vi "UI Main.vi"() -> ()   [LabVIEW 2020]
uses:
  controls/UI Data.ctl
  support/Message Queue/Message Cluster.ctl
  Globals/Global - All UI Loop Stop.vi
  Globals/Global - UI Stream and Variable Connections.vi
  Globals/Global - Configuration Options.vi
  support/User Event - Stop/User Event - Stop.lvlib
  support/Message Queue/Message Queue.lvlib
panel:
  in  "UI Error":string="UI Error"
  in  "Invalid Message Loop Message":string="The invalid message string \"%s\" was received in the Message Handling Loop."
  out "Current Logging State":u16(ring) items=["Logging", "Idle (Safe State)", "Unknown - Disconnected"]
  in  "Exit":bool
  out "System Status":string
  in  "Settings Tab":enum32{"UI Commands", "System Monitoring"}(tab)
  in  "Live Data Channel":u32 max=3 step=1
  out "Live Data":waveform(dbl)(graph)
  in  "Stop Live Data":bool
  in  "Acquire Live Data":bool
  out "Most recent manually-triggered log file":path
  in  "Force Trigger":bool
  out "Number of Data Files":u32
  out "Largest Contiguous Memory (bytes)":dbl(graph)
  out "Resource Utilization (%)":cluster{dbl, "Double":dbl, dbl}(graph)
  out "System Time":timestamp
  out "Connected?":bool
  in  "Connect to Controller":bool
  in  "Controller Address":string
  # "LabVIEW Real-Time Waveform Acquisition and Logging (NI-DAQmx)"
  # "Connection Settings"
  # "Live Data"
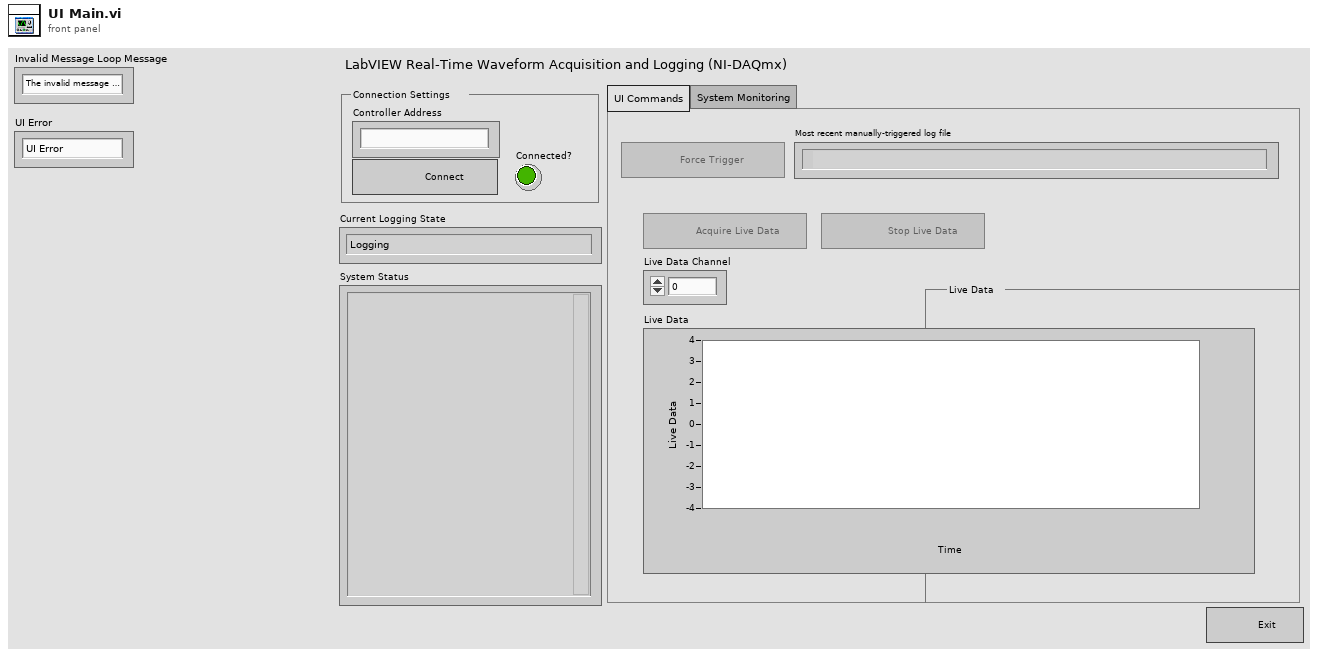
[diagram p1: front panel]
types:
  T1 = typedef "UI Data.ctl" = cluster{"Create Log File Ref":refnum<vi>, "Acquire Live Data Ref":refnum<vi>, "Stop Live Data Ref":refnum<vi>}
  T2 = typedef "Message Queue.lvlib/All Host Message Queues.ctl" = cluster{"UI":refnum<queue>}
  T3 = typedef "Message Queue.lvlib/Message Cluster.ctl" = cluster{"Message":string, "Message Data":variant}
  T4 = typedef "Variable References.ctl" = cluster{"CPU Usage":refnum<k21>, "Contiguous Memory":refnum<k21>, "Buffer Backlog":refnum<k21>, "Drive Space":refnum<k21>, "Number of Data Files":refnum<k21>, "System Time":refnum<k21>}
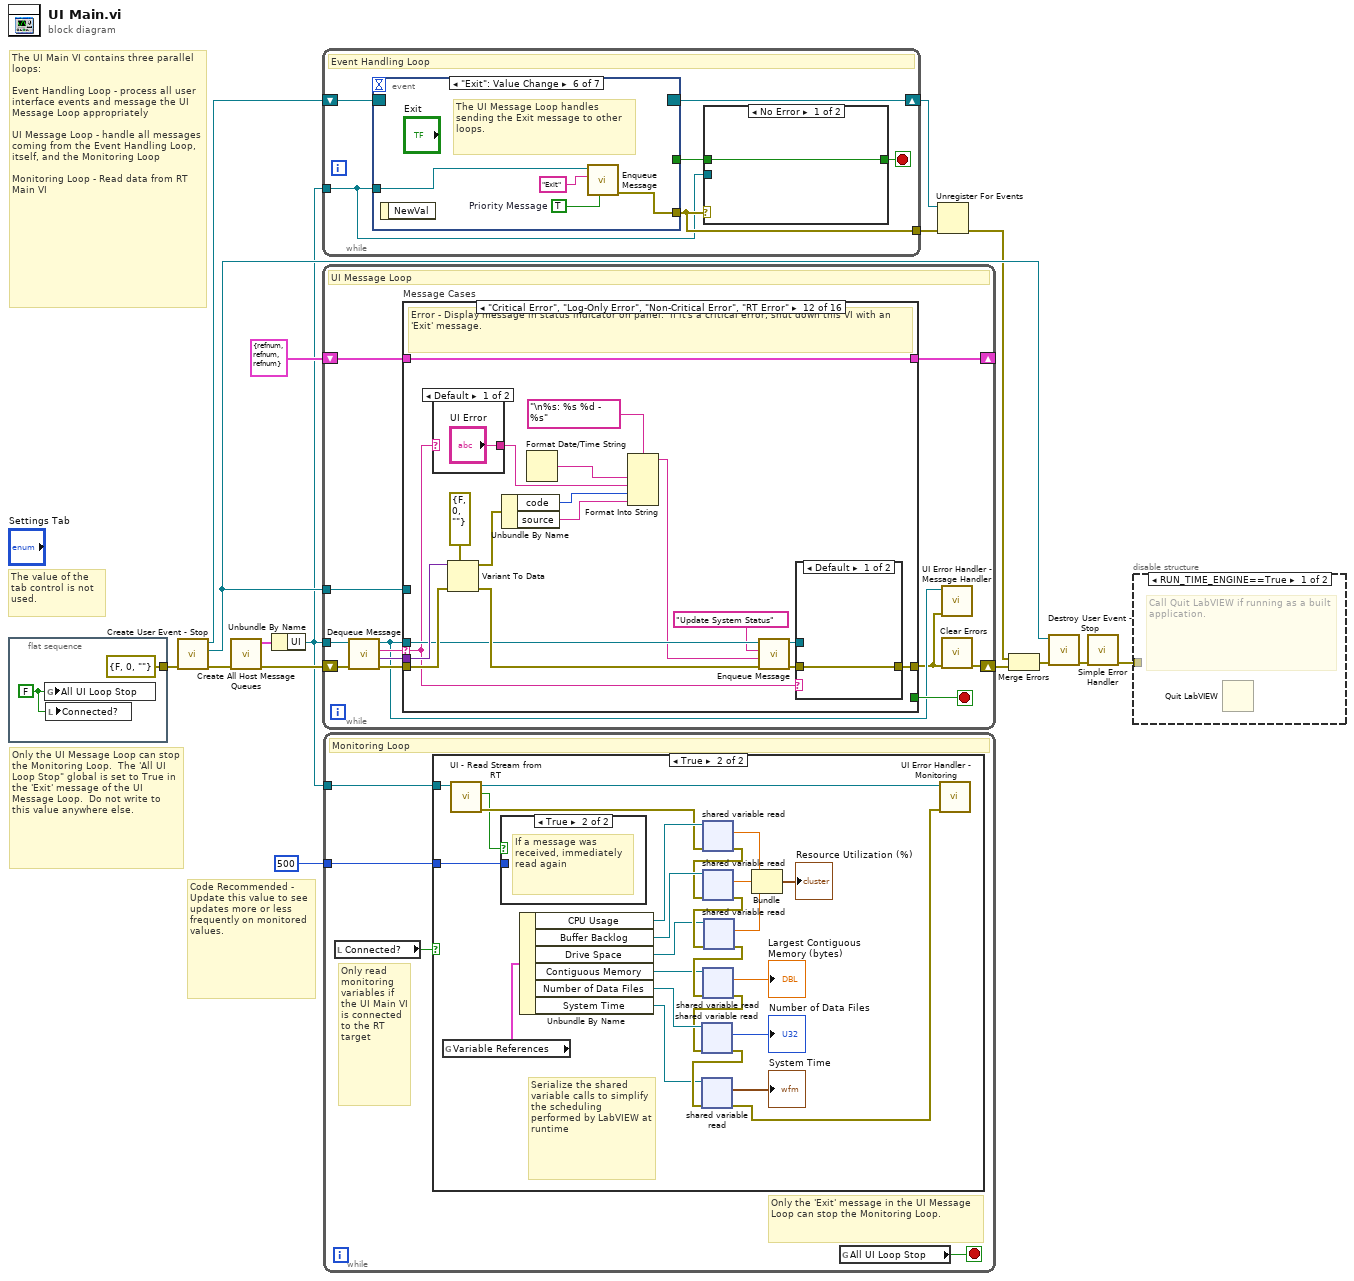
[diagram p0: block diagram]
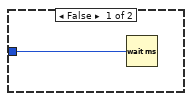
[diagram p3: hidden frame]
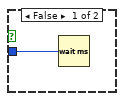
[diagram p4: hidden frame]
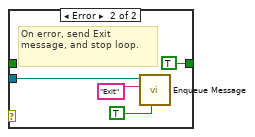
[diagram p5: hidden frame]
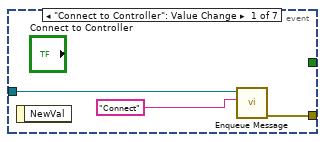
[diagram p6: hidden frame]
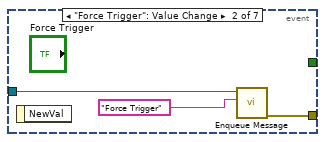
[diagram p7: hidden frame]
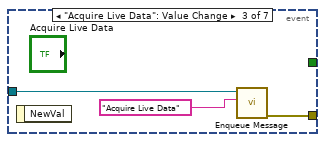
[diagram p8: hidden frame]
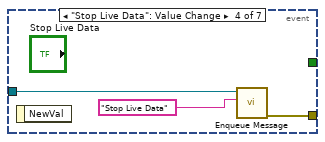
[diagram p9: hidden frame]
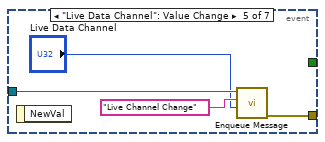
[diagram p10: hidden frame]
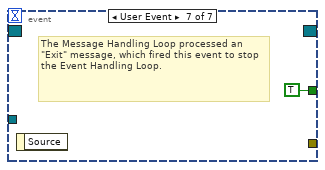
[diagram p11: hidden frame]
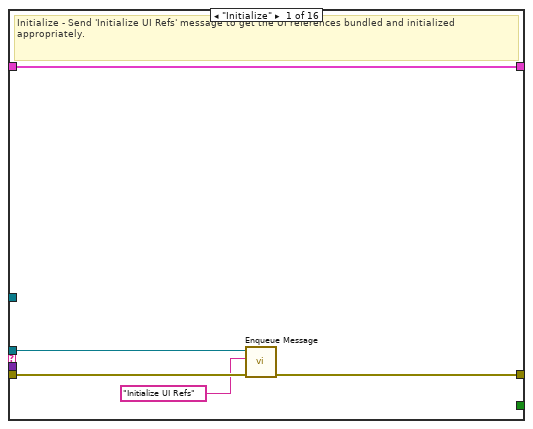
[diagram p12: hidden frame]
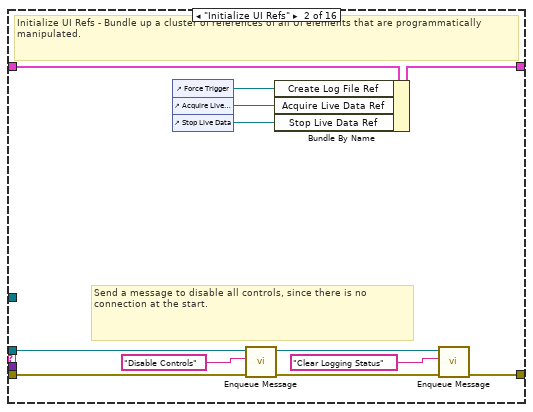
[diagram p13: hidden frame]
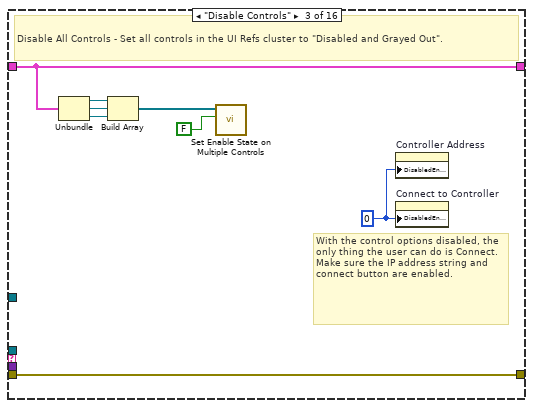
[diagram p14: hidden frame]
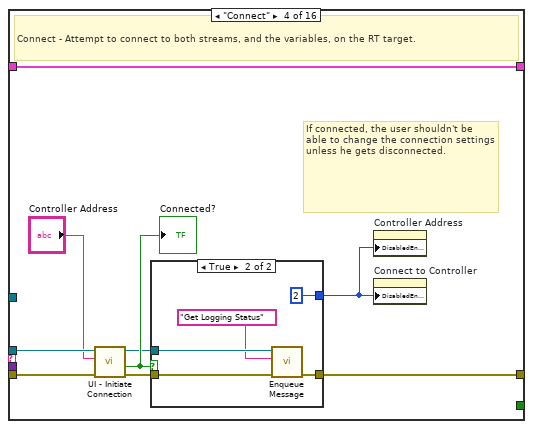
[diagram p15: hidden frame]
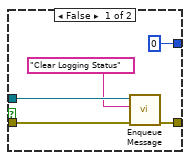
[diagram p16: hidden frame]
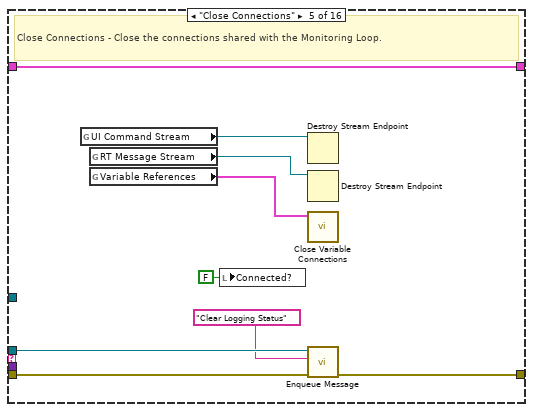
[diagram p17: hidden frame]
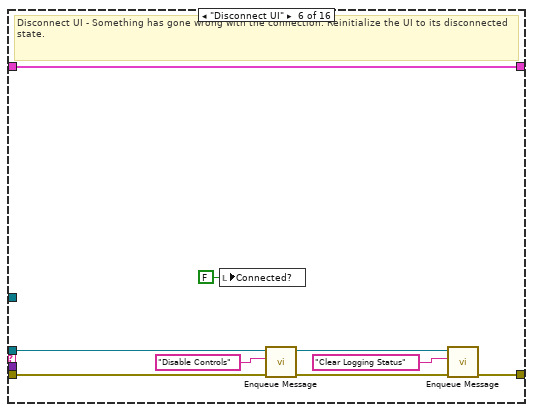
[diagram p18: hidden frame]
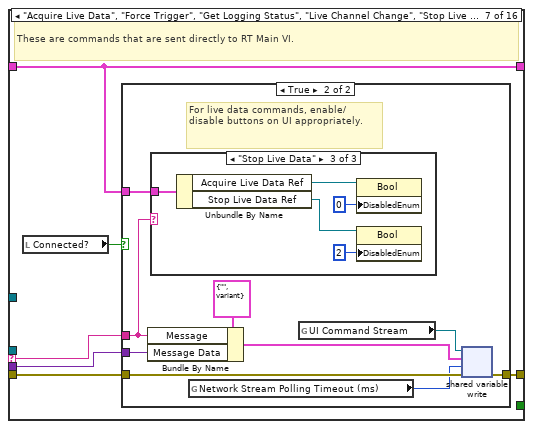
[diagram p19: hidden frame]
diagram:
  # "Code Recommended - Update this value to see updates more or less frequently on monitored values."
  # "The UI Main VI contains three parallel loops:\n\nEvent Handling Loop - process all user interface events and message the UI Message Loop appropriately\n\nUI Message Loop - handle all messages coming from the Event Handling Loop, itself, and the Monitoring Loop\n\nMonitoring Loop - Read data from RT Main VI"
  # "The value of the tab control is not used."
  # "Only the UI Message Loop can stop the Monitoring Loop.  The 'All UI Loop Stop\" global is set to True in the 'Exit' message of the UI Message Loop.  Do not write to this value anywhere else."
  n1 = flat-sequence {
    tunnel: [errorcluster {"status"=FALSE, "code"=0, "source"=""} ("error in (no error)")] -> w3
    frame #0 {
      w17 = FALSE
      n2 = global write "Global - All UI Loop Stop.vi" "All UI Loop Stop"(w17) -> ()
      n3 = local write "Connected?"(w17) -> ()
    }
  }
  n4 = call "Create User Event - Stop.vi"("error in (no error)"=w3) -> ("error out"=w11:errorcluster, "User Event - Stop"=w12:refnum<user-event>, "Stop Event Registration Refnum"=w13:refnum<event-registration>)  [unwired: 8 in]
  n5 = call "Create All Host Message Queues.vi"("error in (no error)"=w11) -> ("error out"=w9:errorcluster, "Message Queues out"=w10:T2)  [unwired: 9 in]
  n6 = Unbundle By Name(w10) -> ("UI"=w4:refnum<queue>)
  n7 = while {
    tunnel: w4 -> [w20]
    tunnel: [w22] -> w15
    shift-right: [w19] -> w7
    shift-left: w13 -> [w21]
    stop <- w23 stop-if-true
    # "Event Handling Loop"
    n8 = event shown="[5] \"Exit\": Value Change" {
      selector: w21 -> [_ _ _ _ _ _ _]
      dyn-events: [_ _ _ _ _ _ _] -> w19
      timeout: _ -> [_ _ _ _ _ _ _]
      tunnel: [_ _ _ _ _ _ TRUE ("Discard?")] -> w24
      tunnel: w20 -> [w30 w33 w36 w39 w43 w46 _]
      tunnel: [w32 w35 w38 w41 w45 w49 _] -> w22
      event "Connect to Controller": Value Change {
        n9 = event-data() -> ()  [unwired: 1 in, 1 out]
        n10 = call "Enqueue Message.vi"("Message"="Connect", "Message Queue"=w30) -> ("error out"=w32:errorcluster)  [unwired: 8 in, 1 out]
      }
      event "Force Trigger": Value Change {
        n11 = event-data() -> ()  [unwired: 1 in, 1 out]
        n12 = call "Enqueue Message.vi"("Message"="Force Trigger", "Message Queue"=w33) -> ("error out"=w35:errorcluster)  [unwired: 8 in, 1 out]
      }
      event "Acquire Live Data": Value Change {
        n13 = event-data() -> ()  [unwired: 1 in, 1 out]
        n14 = call "Enqueue Message.vi"("Message"="Acquire Live Data", "Message Queue"=w36) -> ("error out"=w38:errorcluster)  [unwired: 8 in, 1 out]
      }
      event "Stop Live Data": Value Change {
        n15 = event-data() -> ()  [unwired: 1 in, 1 out]
        n16 = call "Enqueue Message.vi"("Message"="Stop Live Data", "Message Queue"=w39) -> ("error out"=w41:errorcluster)  [unwired: 8 in, 1 out]
      }
      event "Live Data Channel": Value Change {
        n17 = event-data() -> ()  [unwired: 1 in, 1 out]
        n18 = call "Enqueue Message.vi"("Message Data"="Live Data Channel", "Message"="Live Channel Change", "Message Queue"=w43) -> ("error out"=w45:errorcluster)  [unwired: 7 in, 1 out]
      }
      event "Exit": Value Change {
        w47 = TRUE  # Priority Message
        # "The UI Message Loop handles sending the Exit message to other loops."
        n19 = event-data() -> ()  [unwired: 1 in, 1 out]
        n20 = call "Enqueue Message.vi"("Priority Message? (F)"=w47, "Message"="Exit", "Message Queue"=w46) -> ("error out"=w49:errorcluster)  [unwired: 7 in, 1 out]
      }
      event User Event {
        # "The Message Handling Loop processed an \"Exit\" message, which fired this event to stop the Event Handling Loop."
        n21 = event-data() -> ()  [unwired: 1 in, 1 out]
      }
    }
    n22 = case shown="No Error" w22 {
      tunnel: [w25 TRUE ("Discard?")] -> w23
      tunnel: w24 -> [w25 _]
      tunnel: w20 -> [_ w26]
      frame No Error {
      }
      frame Error {
        # "On error, send Exit message, and stop loop."
        n23 = call "Enqueue Message.vi"("Priority Message? (F)"=TRUE ("Discard?"), "Message"="Exit", "Message Queue"=w26) -> ()  [unwired: 7 in, 2 out]
      }
    }
  }
  n24 = while {
    tunnel: w4 -> [w56]
    tunnel: w12 -> [w61]
    shift-right: [w51] -> w16
    shift-left: w9 -> [w60]
    shift-right: [w54] -> _
    shift-left: T1 {"Create Log File Ref"=refnum, "Acquire Live Data Ref"=refnum, "Stop Live Data Ref"=refnum} ("Measurement UI Controls") -> [w55]
    stop <- w62 stop-if-true
    # "UI Message Loop"
    n25 = call "Dequeue Message.vi"("error in (no error)"=w60, "Message Queue"=w56) -> ("error out"=w59:errorcluster, "Message Data"=w57:variant, "Message"=w58:string, "dup Message Queue"=w53:refnum<queue>)  [unwired: 6 in]
    n26 = case "Message Cases" shown="\"Critical Error\", \"Log-Only Error\", \"Non-Critical Error\", \"RT Error\"" w58 {
      selector: w58 -> [_ _ _ _ _ _ w127 _ _ _ _ w182 _ _ _ w244]
      tunnel: w53 -> [w64 w76 _ w95 w108 w121 _ _ _ _ _ w186 _ w229 _ _]
      tunnel: w59 -> [w66 w79 w87 w96 w110 w122 w130 w156 w162 w177 w178 w196 w217 w234 w239 _]
      tunnel: [w65 w69 w87 w90 w109 w118 w129 w154 w160 w176 w178 w197 w215 w235 w238 w242] -> w52
      tunnel: [_ _ _ _ _ _ _ _ _ _ _ _ _ TRUE _ _] -> w62
      tunnel: w57 -> [_ _ _ _ _ _ w128 w153 w159 w175 _ w194 w214 _ _ _]
      tunnel: w61 -> [_ _ _ _ _ _ _ _ _ _ _ _ _ w233 _ _]
      tunnel: w55 -> [w67 w78 w86 w94 w115 w124 w126 w155 w161 w170 w180 w198 w216 w231 w237 w240]
      tunnel: [w67 w77 w86 w94 w115 w124 w126 w155 w161 w170 w180 w198 w216 w231 w237 w240] -> w54
      frame "Initialize" {
        # "Initialize - Send 'Initialize UI Refs' message to get the UI references bundled and initialized appropriately."
        n27 = call "Enqueue Message.vi"("error in (no error)"=w66, "Message"="Initialize UI Refs", "Message Queue"=w64) -> ("error out"=w65:errorcluster)  [unwired: 7 in, 1 out]
      }
      frame "Initialize UI Refs" {
        # "Send a message to disable all controls, since there is no connection at the start."
        # "Initialize UI Refs - Bundle up a cluster of references of all UI elements that are programmatically manipulated."
        n28 = control-ref of="Force Trigger"() -> (w74:refnum<vi>)
        n29 = control-ref of="Acquire Live Data"() -> (w73:refnum<vi>)
        n30 = control-ref of="Stop Live Data"() -> (w72:refnum<vi>)
        n31 = call "Enqueue Message.vi"("error in (no error)"=w79, "Message"="Disable Controls", "Message Queue"=w76) -> ("error out"=w70:errorcluster, "dup Message Queue"=w71:refnum<queue>)  [unwired: 7 in]
        n32 = Bundle By Name(cluster=w78, "Create Log File Ref"=w74, "Acquire Live Data Ref"=w73, "Stop Live Data Ref"=w72) -> (w77:T1)
        n33 = call "Enqueue Message.vi"("error in (no error)"=w70, "Message"="Clear Logging Status", "Message Queue"=w71) -> ("error out"=w69:errorcluster)  [unwired: 7 in, 1 out]
      }
      frame "Disable Controls" {
        w82 = 0
        # "With the control options disabled, the only thing the user can do is Connect. Make sure the IP address string and connect button are enabled."
        # "Disable All Controls - Set all controls in the UI Refs cluster to \"Disabled and Grayed Out\"."
        n34 = Unbundle(w86) -> ("Create Log File Ref"=w85:refnum<vi>, "Acquire Live Data Ref"=w81:refnum<vi>, "Stop Live Data Ref"=w80:refnum<vi>)
        n35 = Build Array(w85, w81, w80) -> (w84:refnum<vi>[])
        n36 = call "Set Enable State on Multiple Controls.vi"("Enable?"=FALSE, "Controls"=w84) -> ()  [unwired: 10 in]
        n37 = property on="Controller Address" class="Str"("DisabledEnum"=w82) -> ()  [unwired: 2 in, 2 out]
        n38 = property on="Connect to Controller" class="Bool"("DisabledEnum"=w82) -> ()  [unwired: 2 in, 2 out]
      }
      frame "Connect" {
        # "If connected, the user shouldn't be able to change the connection settings unless he gets disconnected."
        # "Connect - Attempt to connect to both streams, and the variables, on the RT target."
        n39 = call "UI - Initiate Connection.vi"("error in (no error)"=w96, "Controller Address"="Controller Address", "Message Queue"=w95) -> ("error out"=w92:errorcluster, "Connected?"=w91:bool, "dup Message Queue"=w89:refnum<queue>)  [unwired: 6 in]
        "Connected?" <- w91
        n40 = case shown="True" w91 {
          tunnel: w92 -> [w99 w105]
          tunnel: [w98 w106] -> w90
          tunnel: w89 -> [w100 w104]
          tunnel: [0 2] -> w88
          frame False {
            n41 = call "Enqueue Message.vi"("error in (no error)"=w99, "Message"="Clear Logging Status", "Message Queue"=w100) -> ("error out"=w98:errorcluster)  [unwired: 7 in, 1 out]
          }
          frame True {
            n42 = call "Enqueue Message.vi"("error in (no error)"=w105, "Message"="Get Logging Status", "Message Queue"=w104) -> ("error out"=w106:errorcluster)  [unwired: 7 in, 1 out]
          }
        }
        n43 = property on="Controller Address" class="Str"("DisabledEnum"=w88) -> ()  [unwired: 2 in, 2 out]
        n44 = property on="Connect to Controller" class="Bool"("DisabledEnum"=w88) -> ()  [unwired: 2 in, 2 out]
      }
      frame "Close Connections" {
        # "Close Connections - Close the connections shared with the Monitoring Loop."
        n45 = global read "Global - UI Stream and Variable Connections.vi" "UI Command Stream"() -> (w114:refnum<k21>)
        n46 = global read "Global - UI Stream and Variable Connections.vi" "RT Message Stream"() -> (w113:refnum<k21>)
        n47 = global read "Global - UI Stream and Variable Connections.vi" "Variable References"() -> (w112:T4)
        n48 = local write "Connected?"(FALSE ("Connected?")) -> ()
        n49 = Destroy Stream Endpoint(11:w114) -> ()  [unwired: 1 in, 1 out]
        n50 = Destroy Stream Endpoint(11:w113) -> ()  [unwired: 1 in, 1 out]
        n51 = call "Close Variable Connections.vi"("Variable References"=w112) -> ()  [unwired: 11 in]
        n52 = call "Enqueue Message.vi"("error in (no error)"=w110, "Message"="Clear Logging Status", "Message Queue"=w108) -> ("error out"=w109:errorcluster)  [unwired: 7 in, 1 out]
      }
      frame "Disconnect UI" {
        # "Disconnect UI - Something has gone wrong with the connection. Reinitialize the UI to its disconnected state."
        n53 = local write "Connected?"(FALSE ("Connected?")) -> ()
        n54 = call "Enqueue Message.vi"("error in (no error)"=w122, "Message"="Disable Controls", "Message Queue"=w121) -> ("error out"=w119:errorcluster, "dup Message Queue"=w117:refnum<queue>)  [unwired: 7 in]
        n55 = call "Enqueue Message.vi"("error in (no error)"=w119, "Message"="Clear Logging Status", "Message Queue"=w117) -> ("error out"=w118:errorcluster)  [unwired: 7 in, 1 out]
      }
      frame "Acquire Live Data", "Force Trigger", "Get Logging Status", "Live Channel Change", "Stop Live Data" {
        # "These are commands that are sent directly to RT Main VI."
        n56 = local read "Connected?"() -> (w125:bool)
        n57 = case shown="True" w125 {
          tunnel: w130 -> [w131 w140]
          tunnel: [w131 w139] -> w129
          tunnel: w128 -> [_ w134]
          tunnel: w127 -> [_ w132]
          tunnel: w126 -> [_ w133]
          frame False {
            # "Don't bother trying to send a message to the RT system if UI Main VI isn't even connected"
          }
          frame True {
            # "For live data commands, enable/disable buttons on UI appropriately."
            n58 = Bundle By Name(cluster=T3 {"Message"="", "Message Data"=variant} ("Message Cluster"), "Message"=w132, "Message Data"=w134) -> (w135:T3)
            n59 = case shown="\"Stop Live Data\"" w132 {
              tunnel: w133 -> [_ w145 w150]
              frame Default {
              }
              frame "Acquire Live Data" {
                n60 = Unbundle By Name(w145) -> ("Acquire Live Data Ref"=w144:refnum<vi>, "Stop Live Data Ref"=w143:refnum<vi>)
                n61 = property class="Bool"(reference=w144, "DisabledEnum"=u8 2) -> ()  [unwired: 1 in, 2 out]
                n62 = property class="Bool"(reference=w143, "DisabledEnum"=u8 0) -> ()  [unwired: 1 in, 2 out]
              }
              frame "Stop Live Data" {
                n63 = Unbundle By Name(w150) -> ("Acquire Live Data Ref"=w149:refnum<vi>, "Stop Live Data Ref"=w148:refnum<vi>)
                n64 = property class="Bool"(reference=w149, "DisabledEnum"=u8 0) -> ()  [unwired: 1 in, 2 out]
                n65 = property class="Bool"(reference=w148, "DisabledEnum"=u8 2) -> ()  [unwired: 1 in, 2 out]
              }
            }
            n66 = global read "Global - Configuration Options.vi" "Network Stream Polling Timeout (ms)"() -> (w137:i32)
            n67 = global read "Global - UI Stream and Variable Connections.vi" "UI Command Stream"() -> (w138:refnum<k21>)
            n68 = shared-variable-write(w138, w140, w135, w137) -> (w139:errorcluster)  [unwired: 2 out]
          }
        }
      }
      frame "Send Path to UI" {
        # "Send Path to UI - Message from the RT Main VI containing the path to the manually-triggered log file."
        n69 = Variant To Data(error in=w156, type=path "", Variant=w153) -> (data=→"Most recent manually-triggered log file":path, error out=w154:errorcluster)
      }
      frame "Send Live Data to UI" {
        # "Send Live Data to UI - Message from the RT Main VI containing the latest live data for the specified channel."
        n70 = Variant To Data(error in=w162, type=waveform(dbl) {"t0"=timestamp(0 s since 1904-01-01), "dt"=1.0, "Y"=[]}, Variant=w159) -> (data=→"Live Data":waveform(dbl), error out=w160:errorcluster)
      }
      frame "Send Logging Status" {
        # "TRUE: Logging Normally\nFALSE: Idle (Safe State)"
        # "Send Logging Status - Message from the RT Main VI indicating whether or not logging is happening normally, or if the logging loop is in safe mode."
        n71 = Unbundle By Name(w170) -> ("Create Log File Ref"=w169:refnum<vi>, "Acquire Live Data Ref"=w168:refnum<vi>, "Stop Live Data Ref"=w164:refnum<vi>)
        n72 = Variant To Data(error in=w177, type=FALSE, Variant=w175) -> (data=w165:bool, error out=w176:errorcluster)
        n73 = Build Array(w169, w168) -> (w167:refnum<vi>[])
        n74 = Build Array(w164) -> (w166:refnum<vi>[])
        n75 = Select(t=u16 0, s=w165, f=u16 1) -> (s? t:f=→"Current Logging State":u16)
        n76 = call "Set Enable State on Multiple Controls.vi"("Enable?"=w165, "Controls"=w167) -> ()  [unwired: 10 in]
        n77 = call "Set Enable State on Multiple Controls.vi"("Enable?"=FALSE, "Controls"=w166) -> ()  [unwired: 10 in]
      }
      frame "Clear Logging Status" {
        # "Clear Logging Status - Show nothing when we are not connected to the RT target and therefore cannot be in a logging or safe mode state."
        n78 = local write "Current Logging State"(u16 2) -> ()
      }
      frame "Critical Error", "Log-Only Error", "Non-Critical Error", "RT Error" {
        # "Error - Display message in status indicator on panel.  If it's a critical error, shut down this VI with an 'Exit' message."
        n79 = case shown="Default" w182 {
          selector: w182 -> [_ w200]
          tunnel: ["UI Error" w200] -> w181
          frame Default {
          }
          frame "RT Error" {
          }
        }
        n80 = Variant To Data(error in=w196, type=errorcluster {"status"=FALSE, "code"=0, "source"=""} ("error constant"), Variant=w194) -> (data=w189:errorcluster, error out=w195:errorcluster)
        n81 = Unbundle By Name(w189) -> ("code"=w188:i32, "source"=w192:string)
        n82 = Format Date/Time String() -> (date/time string=w191:string)  [unwired: 3 in]
        n83 = Format Into String(format string="\n%s: %s %d - %s", w191, w181, w188, w192) -> (resulting string=w183:string)  [unwired: 2 in, 1 out]
        n84 = call "Enqueue Message.vi"("error in (no error)"=w195, "Message Data"=w183, "Message"="Update System Status", "Message Queue"=w186) -> ("error out"=w187:errorcluster, "dup Message Queue"=w185:refnum<queue>)  [unwired: 6 in]
        n85 = case shown="Default" w182 {
          tunnel: w187 -> [w201 w205]
          tunnel: w185 -> [_ w203]
          tunnel: [w201 w204] -> w197
          frame Default {
          }
          frame "Critical Error" {
            n86 = call "Enqueue Message.vi"("error in (no error)"=w205, "Message"="Exit", "Message Queue"=w203) -> ("error out"=w204:errorcluster)  [unwired: 7 in, 1 out]
          }
        }
      }
      frame "Update System Status" {
        # "Code Recommended - The code below ensures that the System Status string value does not become too large.  It uses the same maximum size as the RT error log to determine whether or not to remove the last half of the log string. Change this logic if you wish to maintain more/less of the information in the System Status string."
        # "Update System Status - Add a new string to the beginning of the System Status string on the UI."
        n87 = Variant To Data(error in=w217, type="", Variant=w214) -> (data=w211:string, error out=w215:errorcluster)
        n88 = global read "Global - Configuration Options.vi" "Error Log Max Size (bytes)"() -> (w207:i64)
        n89 = local read "System Status"() -> (w209:string)
        n90 = String Length(string=w209) -> (length=w210:i32)
        n91 = Greater?(x=w210, y=w207) -> (0:w208:bool)
        n92 = case shown="True" w208 {
          tunnel: w209 -> [w218 w222]
          tunnel: w207 -> [_ w221]
          tunnel: [w218 w223] -> w206
          frame False {
          }
          frame True {
            n93 = Divide(x=w221, y=i64 2) -> (x/y=w220:dbl)
            n94 = String Subset(string=w222, length (rest)=w220) -> (substring=w223:string)  [unwired: 1 in]
          }
        }
        n95 = Concatenate Strings(w211, w206) -> (→"System Status":string)
      }
      frame "Exit" {
        # "Flush the Writer Stream to ensure all pending messages are sent to RT Main VI"
        # "Close all connections"
        # "Stop Monitoring Loop"
        # "Stop Event Handling Loop"
        # "Release the UI Message queue reference"
        # "Stop UI Message Loop"
        # "Exit - Fire the User Event to stop the Event Handling Loop, and toggle the local variable to stop the Monitoring Loop.  This message alone causes all three loops to stop."
        n96 = global write "Global - All UI Loop Stop.vi" "All UI Loop Stop"(TRUE ("Stop Monitoring Loop")) -> ()
        n97 = call "Fire User Event - Stop.vi"("User Event - Stop"=w233) -> ("error out"=w232:errorcluster)  [unwired: 10 in]
        n98 = Release Queue(queue=w229, error in (no error)=w234) -> (error out=w230:errorcluster)  [unwired: 1 in, 2 out]
        n99 = global read "Global - UI Stream and Variable Connections.vi" "UI Command Stream"() -> (w225:refnum<k21>)
        n100 = global read "Global - UI Stream and Variable Connections.vi" "RT Message Stream"() -> (w227:refnum<k21>)
        n101 = global read "Global - UI Stream and Variable Connections.vi" "Variable References"() -> (w226:T4)
        n102 = Flush Stream(11:w225) -> (3:w224:refnum<k21>)  [unwired: 3 in, 2 out]
        n103 = Destroy Stream Endpoint(11:w224) -> ()  [unwired: 1 in, 1 out]
        n104 = Destroy Stream Endpoint(11:w227) -> ()  [unwired: 1 in, 1 out]
        n105 = call "Close Variable Connections.vi"("Variable References"=w226) -> ()  [unwired: 11 in]
        n106 = Merge Errors(w232, w230) -> (w235:errorcluster)
      }
      frame "---Copy This Frame---" {
        # "Duplicate this frame when creating new messages.  Change this comment in the duplicated frame to describe this message."
        n107 = Merge Errors(w239) -> (w238:errorcluster)
      }
      frame Default {
        # "'Default' case only runs if there is a message that isn't defined in any of the other cases.  Output a programming error."
        n108 = Format Into String(format string="Invalid Message Loop Message", w244) -> (resulting string=w241:string)  [unwired: 2 in, 1 out]
        n109 = call <vilib>:"Error Cluster From Error Code.vi"("error message (\"\")"=w241, "error code (0)"=1) -> ("error out"=w242:errorcluster)  [unwired: 7 in]
      }
    }
    n110 = call "UI Error Handler - Message Handler.vi"("error in (no error)"=w52, "Message Queue"=w53) -> ()  [unwired: 9 in, 1 out]
    n111 = call <vilib>:"Clear Errors.vi"("error in (no error)"=w52) -> ("error out"=w51:errorcluster)  [unwired: 5 in, 1 out]
  }
  n112 = while {
    tunnel: w4 -> [w248]
    tunnel: u32 500 ("milliseconds to wait") -> [w246]
    stop <- w249 stop-if-true
    # "Only read monitoring variables if the UI Main VI is connected to the RT target"
    # "Only the 'Exit' message in the UI Message Loop can stop the Monitoring Loop."
    # "Monitoring Loop"
    n113 = local read "Connected?"() -> (w247:bool)
    n114 = case shown="True" w247 {
      tunnel: w248 -> [_ w272]
      tunnel: w246 -> [w250 w252]
      frame False {
        n115 = Wait (ms)(milliseconds to wait=w250) -> ()  [unwired: 1 out]
      }
      frame True {
        # "Serialize the shared variable calls to simplify the scheduling performed by LabVIEW at runtime"
        n116 = global read "Global - UI Stream and Variable Connections.vi" "Variable References"() -> (w270:T4)
        n117 = call "UI - Read Stream from RT.vi"("Message Queue"=w272) -> ("error out"=w273:errorcluster, "Message Received?"=w253:bool, "dup Message Queue"=w271:refnum<queue>)  [unwired: 8 in]
        n118 = case shown="True" w253 {
          tunnel: w252 -> [w276 _]
          frame False {
            n119 = Wait (ms)(milliseconds to wait=w276) -> ()  [unwired: 1 out]
          }
          frame True {
            # "If a message was received, immediately read again"
          }
        }
        n120 = Unbundle By Name(w270) -> ("CPU Usage"=w275:refnum<k21>, "Buffer Backlog"=w274:refnum<k21>, "Drive Space"=w254:refnum<k21>, "Contiguous Memory"=w262:refnum<k21>, "Number of Data Files"=w259:refnum<k21>, "System Time"=w255:refnum<k21>)
        n121 = shared-variable-read(w275, w273) -> (w269:errorcluster, w267:dbl)  [unwired: 2 out]
        n122 = shared-variable-read(w274, w269) -> (w268:errorcluster, w266:dbl)  [unwired: 2 out]
        n123 = shared-variable-read(w254, w268) -> (w263:errorcluster, w265:dbl)  [unwired: 2 out]
        n124 = shared-variable-read(w262, w263) -> (w251:errorcluster, →"Largest Contiguous Memory (bytes)":dbl)  [unwired: 2 out]
        n125 = shared-variable-read(w259, w251) -> (w258:errorcluster, →"Number of Data Files":u32)  [unwired: 2 out]
        n126 = shared-variable-read(w255, w258) -> (w256:errorcluster, →"System Time":timestamp)  [unwired: 2 out]
        n127 = Bundle(w267, "Double"=w266, w265) -> (→"Resource Utilization (%)":cluster{dbl, "Double":dbl, dbl})  [unwired: 1 in]
        n128 = call "UI Error Handler - Monitoring.vi"("error in (no error)"=w256, "Message Queue"=w271) -> ()  [unwired: 9 in, 1 out]
      }
    }
    n129 = global read "Global - All UI Loop Stop.vi" "All UI Loop Stop"() -> (w249:bool)
  }
  n130 = Unregister For Events(event registration refnum=w7, error in=w15) -> (error out=w8:errorcluster)
  n131 = Merge Errors(w8, w16) -> (w14:errorcluster)
  n132 = call "Destroy User Event - Stop.vi"("error in (no error)"=w14, "User Event - Stop"=w12) -> ("error out"=w5:errorcluster)  [unwired: 9 in]
  n133 = call <vilib>:"Simple Error Handler.vi"("error in (no error)"=w5) -> ("error out"=w1:errorcluster)  [unwired: 4 in, 4 out]
  n134 = disable-structure shown="RUN_TIME_ENGINE==True" {
    disable-tunnel: w1 -> [_ _]
    frame condition #0 {
      # "Call Quit LabVIEW if running as a built application."
      n135 = Quit LabVIEW() -> ()  [unwired: 1 in]
    }
    frame condition #1 (active) {
    }
  }
